vi "Actor Core.vi"(8 "error in":errorcluster caption="错误输入", 11 "GlobalPlannerPyPl in":refnum<class "GlobalPlannerPyPl.lvclass"> caption="操作者输入") -> (0 "error out":errorcluster caption="错误输出", 3 "Actor out":refnum<class "Actor.lvclass"> caption="操作者输出")   [LabVIEW 2014, in "GlobalPlannerPyPl.lvlib" / "GlobalPlannerPyPl.lvclass"]
doc: "(<B>文件名</B>：Actor Framework.lvlib:Actor.lvclass:Actor Core.vi)\n\n接收发送至操作者的消息，响应消息并处理可能导致操作者关闭的错误。\n\n子孙类重写该VI，使操作者完成特定的任务。使用调用父方法节点实现重写。"
uses:
  GlobalPlannerPyPl.lvclass
  <vilib>/ActorFramework/Actor/Actor.lvclass
  <vilib>/ActorFramework/Actor/Actor.lvclass/Actor.ctl
  GlobalPlannerPyPl.lvclass/GlobalPlannerPyPl.ctl
  <vilib>/ActorFramework/Message Enqueuer/Message Enqueuer.lvclass/Message Enqueuer.ctl
  <vilib>/ActorFramework/Message Enqueuer/Enqueue.vi
  <vilib>/ActorFramework/Message Priority Queue/Priority Enqueue.vi
  Global_var/Global_var.vi
  Wrapper_lib/zsActor/ActorWrapper.lvclass
panel:
  out "goal_with_force_array":T1(array[cluster])
  out "GlobalPlanner_Recycle":bool
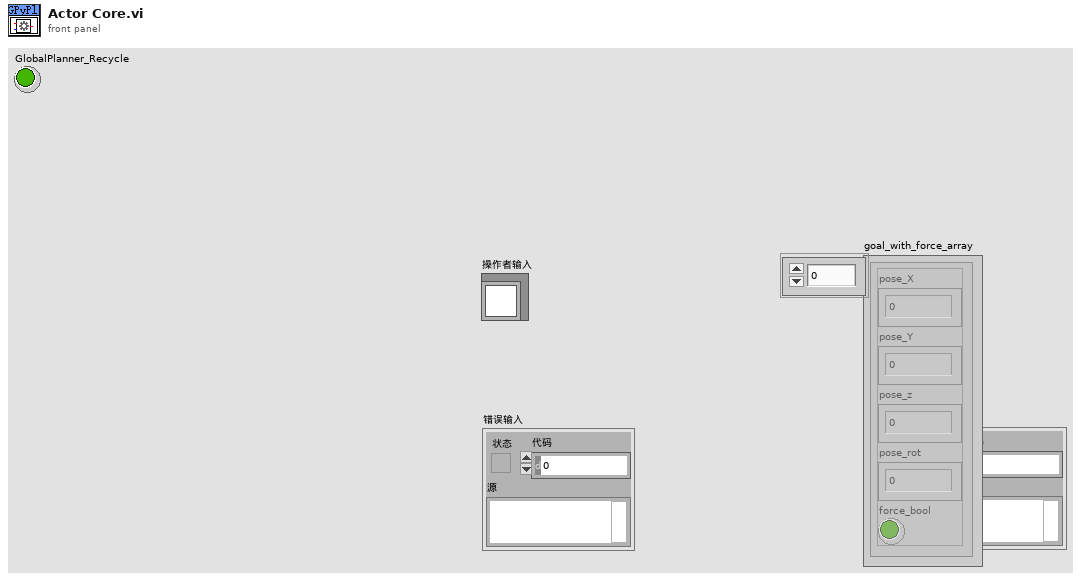
[diagram p1: front panel]
types:
  T1 = cluster{"pose_X":dbl, "pose_Y":dbl, "pose_z":dbl, "pose_rot":dbl, "force_bool":bool}[]
  T2 = cluster{"pose_X":dbl, "pose_Y":dbl, "pose_z":dbl, "pose_rot":dbl, "force_bool":bool}
  T3 = cluster{"now_pose_X":dbl, "now_pose_Y":dbl, "now_pose_Rot_deg":dbl}
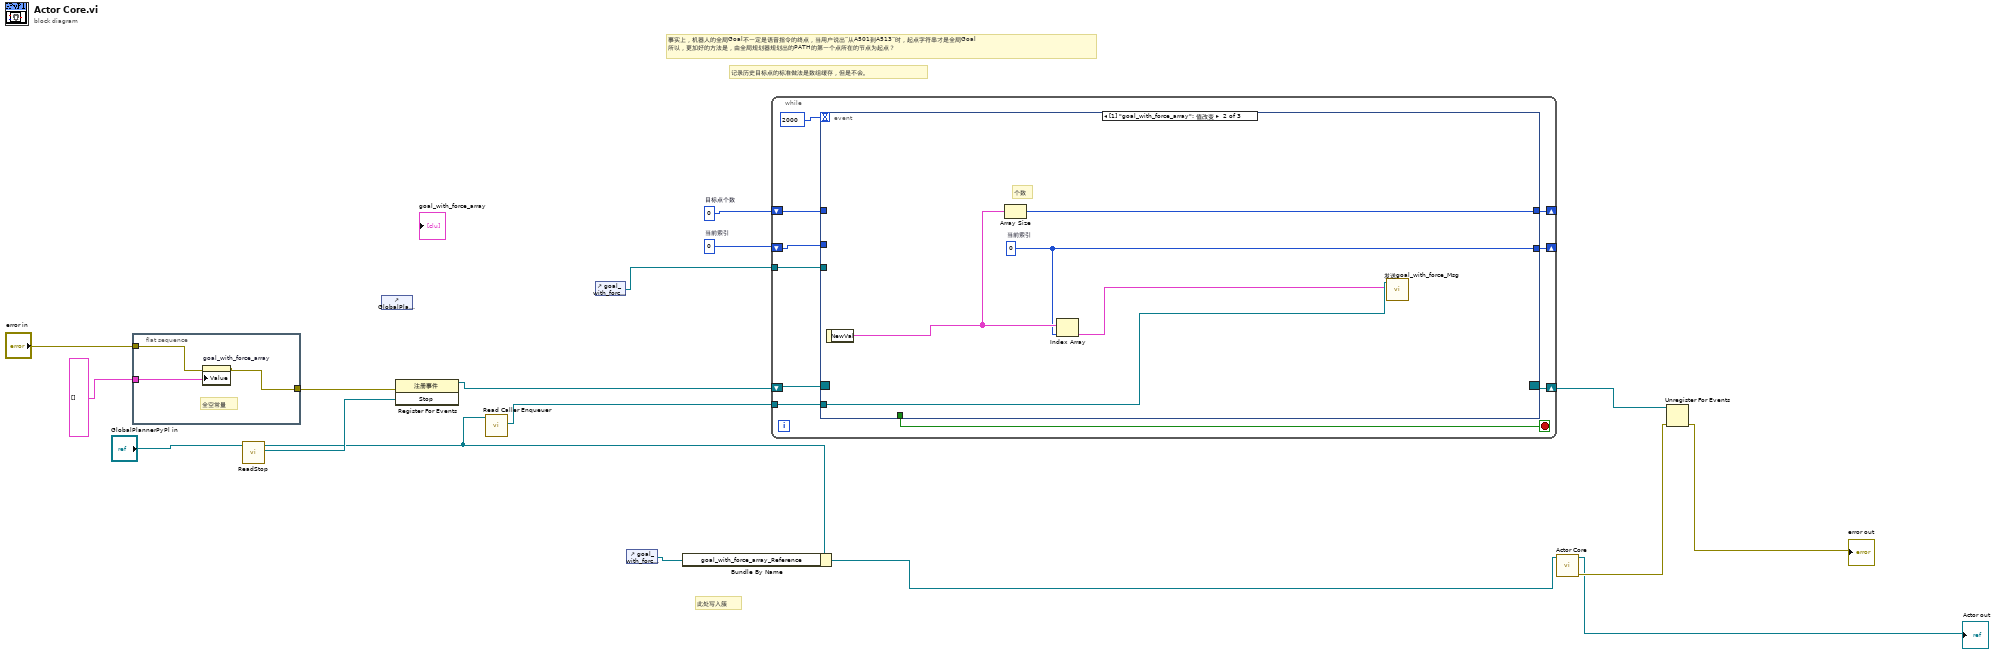
[diagram p0: block diagram]
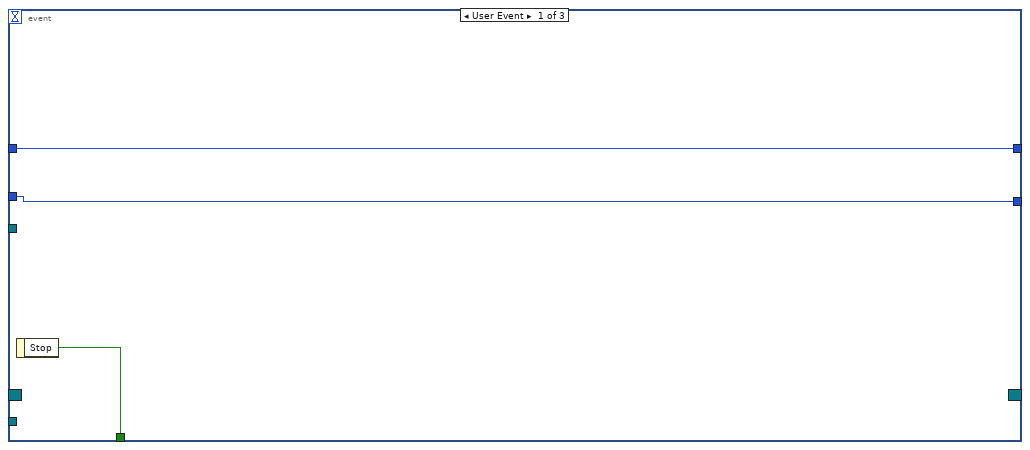
[diagram p2: hidden frame]
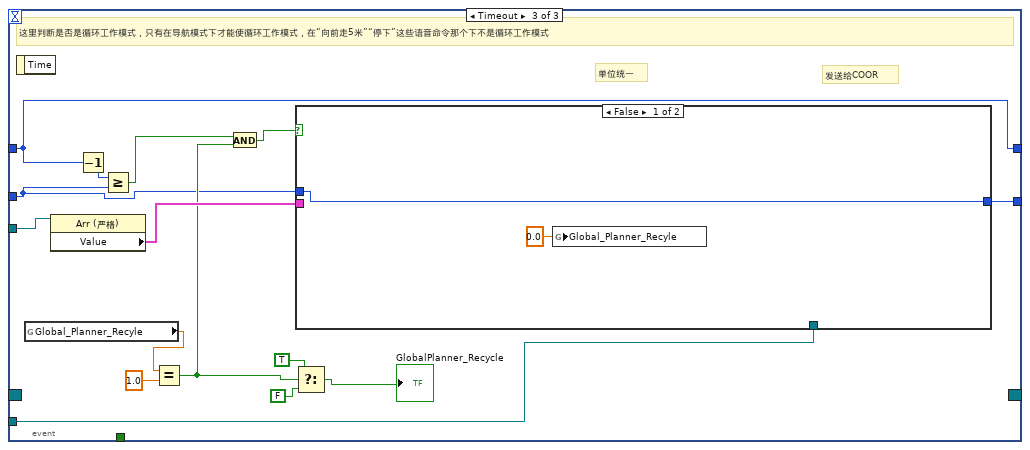
[diagram p3: hidden frame]
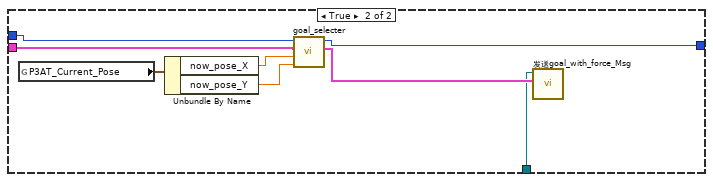
[diagram p4: hidden frame]
diagram:
  w2 = 0  # 当前索引
  w1 = 0  # 目标点个数
  # "此处写入簇"
  # "记录历史目标点的标准做法是数组缓存，但是不会。"
  # "事实上，机器人的全局Goal不一定是语音指令的终点，当用户说出“从A501到A513”时，起点字符串才是全局Goal\n所以，更加好的方法是，由全局规划器规划出的PATH的第一个点所在的节点为起点？"
  n1 = flat-sequence {
    tunnel: [w19] -> w16
    tunnel: "error in" -> [w20]
    tunnel: T1 [] ("值") -> [w18]
    frame #0 {
      # "全空常量"
      n2 = property on="goal_with_force_array" class="Arr (严格)"(error in=w20, "Value"=w18) -> (error out=w19:errorcluster)  [unwired: 1 in, 1 out]
    }
  }
  n3 = call-dynamic "ReadStop.vi"("zsActor输入"="GlobalPlannerPyPl in") -> ("Stop"=w17:refnum<user-event>, "zsActor输出"=w7:refnum<class "GlobalPlannerPyPl.lvclass">)  [unwired: 8 in, 1 out]
  n4 = control-ref of="GlobalPlanner_Recycle"() -> ()  [unwired: 1 out]
  n5 = register-events(error in=w16, w17) -> (reference out=w14:refnum<event-registration>)  [unwired: 1 in, 1 out]
  n6 = call <vilib>:"Read Caller Enqueuer.vi"("Actor"=w7) -> ("Caller Enqueuer"=w15:refnum<class "Message Enqueuer.lvclass">)  [unwired: 10 in]
  n7 = control-ref of="goal_with_force_array"() -> (w4:refnum<vi>)
  n8 = control-ref of="goal_with_force_array"() -> (w5:refnum<vi>)
  n9 = Bundle By Name(cluster=w7, "goal_with_force_array_Reference"=w5) -> (w6:refnum<class "GlobalPlannerPyPl.lvclass">)
  n10 = while {
    tunnel: w15 -> [w30]
    shift-right: [w28] -> w13
    shift-left: w14 -> [w29]
    tunnel: w4 -> [w25]
    shift-right: [w24] -> _
    shift-left: w1 -> [w22]
    shift-right: [w23] -> _
    shift-left: w2 -> [w21]
    stop <- w27 stop-if-true
    n11 = event shown="[1] \"goal_with_force_array\": 值改变" {
      selector: w29 -> [_ _ _]
      dyn-events: [_ _ _] -> w28
      timeout: 2000 -> [_ _ _]
      tunnel: w30 -> [_ w35 w39]
      tunnel: [w33 _ _] -> w27
      tunnel: w25 -> [_ _ w53]
      tunnel: [w32 w37 w46] -> w24
      tunnel: [w31 w36 w40] -> w23
      tunnel: w22 -> [w32 _ w46]
      tunnel: w21 -> [w31 _ w41]
      event User Event {
        n12 = event-data() -> ("Stop"=w33:bool)  [unwired: 1 in]
      }
      event "goal_with_force_array": Value Change {
        w36 = 0  # 当前索引
        # "个数"
        n13 = event-data() -> ("NewVal"=w38:T1)  [unwired: 1 in]
        n14 = Array Size(array=w38) -> (size(s)=w37:i32)
        n15 = Index Array(array=w38, index=w36) -> (element=w34:T2)
        n16 = call "发送goal_with_force_Msg.vi"("值(信号)"=w34, "消息待入队列"=w35) -> ()  [unwired: 8 in, 2 out]
      }
      event Timeout {
        # "发送给COOR"
        # "单位统一"
        # "这里判断是否是循环工作模式，只有在导航模式下才能使循环工作模式，在“向前走5米”“停下”这些语音命令那个下不是循环工作模式"
        n17 = event-data() -> ()  [unwired: 1 in, 1 out]
        n18 = global read "Global_var.vi" "Global_Planner_Recyle"() -> (w48:dbl)
        n19 = property class="Arr (严格)"(reference=w53) -> ("Value"=w49:T1)  [unwired: 1 in, 2 out]
        n20 = Decrement(x=w46) -> (x-1=w45:i32)
        n21 = Greater Or Equal?(x=w45, y=w41) -> (x >= y?=w44:bool)
        n22 = Equal?(x=w48, y=1.0) -> (x = y?=w43:bool)
        n23 = And(x=w44, y=w43) -> (x .and. y?=w42:bool)
        n24 = case shown="真" w42 {
          tunnel: w49 -> [_ w61]
          tunnel: w41 -> [w55 w62]
          tunnel: [w55 w58] -> w40
          tunnel: w39 -> [_ w56]
          frame False {
            n25 = global write "Global_var.vi" "Global_Planner_Recyle"(0.0 ("Global_Planner_Recyle")) -> ()
          }
          frame True {
            n26 = global read "Global_var.vi" "P3AT_Current_Pose"() -> (w63:T3)
            n27 = Unbundle By Name(w63) -> ("now_pose_X"=w60:dbl, "now_pose_Y"=w59:dbl)
            n28 = call "goal_selecter.vi"("当前索引"=w62, "值"=w61, "now_pose_X"=w60, "now_pose_Y"=w59) -> ("新索引new"=w58:i32, "goal_with_force"=w57:T2)  [unwired: 5 in]
            n29 = call "发送goal_with_force_Msg.vi"("值(信号)"=w57, "消息待入队列"=w56) -> ()  [unwired: 8 in, 2 out]
          }
        }
        n30 = Select(t=TRUE, s=w43, f=FALSE) -> (s? t:f=→"GlobalPlanner_Recycle":bool)
      }
    }
  }
  n31 = call-parent "Actor Core.vi"("Actor in"=w6) -> ("error out"=w12:errorcluster, "Actor out"=→"Actor out":refnum<class "Actor.lvclass">)  [unwired: 9 in]
  n32 = Unregister For Events(event registration refnum=w13, error in=w12) -> (error out=→"error out":errorcluster)
